vi "Configure Tare.vi"(8 "error in (no error)":errorcluster, 9 "Tare Value [g]":dbl, 10 "Set Value (F:Tare with current value)":bool, 11 "VISA resource name":refnum<visa-resource-name>) -> (0 "error out":errorcluster, 3 "VISA resource name out":refnum<visa-resource-name>)   [LabVIEW 2017, in "RadWag balances and scales.lvlib"]
doc: "Configures tare for the balance with current or given weight."
uses:
  <instrlib>/Radwag Balances and Scales/Public/RadWag balances and scales.lvlib
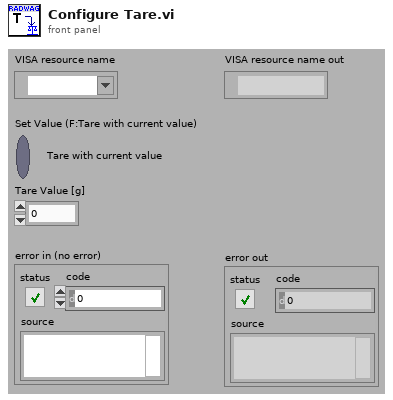
[diagram p1: front panel]
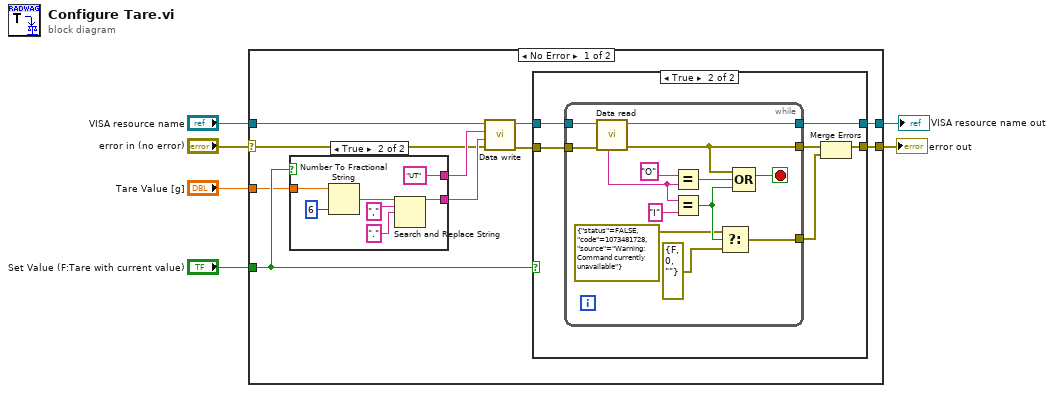
[diagram p0: block diagram]
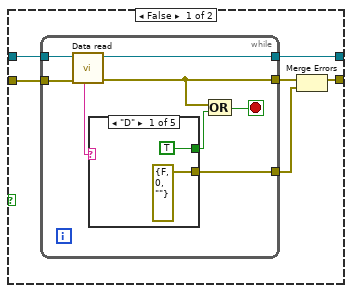
[diagram p2: hidden frame]
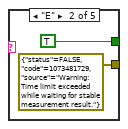
[diagram p3: hidden frame]
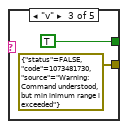
[diagram p4: hidden frame]
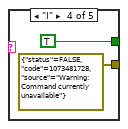
[diagram p5: hidden frame]
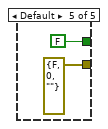
[diagram p6: hidden frame]
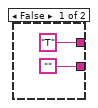
[diagram p7: hidden frame]
diagram:
  n1 = case shown="No Error" "error in (no error)" {
    selector: "error in (no error)" -> [w7 w69]
    tunnel: "VISA resource name" -> [w16 w70]
    tunnel: [w14 w70] -> w5
    tunnel: "Set Value (F:Tare with current value)" -> [w10 _]
    tunnel: [w9 w69] -> w3
    tunnel: "Tare Value [g]" -> [w8 _]
    frame No Error {
      n2 = case shown="True" w10 {
        tunnel: ["T" ("ID") "UT" ("ID")] -> w12
        tunnel: ["" w65] -> w11
        tunnel: w8 -> [_ w62]
        frame False {
        }
        frame True {
          n3 = Number To Fractional String(number=w62, precision (6)=i16 6) -> (F-format string=w66:string)  [unwired: 2 in]
          n4 = Search and Replace String(input string=w66, search string=",", replace string="." ("replace string (\"\")")) -> (result string=w65:string)  [unwired: 5 in, 3 out]
        }
      }
      n5 = call <instrlib>:"Data write.vi"("error in (no error)"=w7, "Parameter"=w11, "ID"=w12, "VISA resource name"=w16) -> ("error out"=w13:errorcluster, "VISA resource name out"=w15:refnum<visa-resource-name>)  [unwired: 6 in]
      n6 = case shown="True" w10 {
        tunnel: w15 -> [w22 w46]
        tunnel: [w20 w44] -> w14
        tunnel: w13 -> [w21 w45]
        tunnel: [w17 w42] -> w9
        frame False {
          n7 = while {
            tunnel: w22 -> [w30]
            tunnel: w21 -> [w29]
            tunnel: [w27] -> w20
            tunnel: [w26] -> w18
            tunnel: [w23] -> w19
            stop <- w28 stop-if-true
            n8 = call <instrlib>:"Data read.vi"("error in (no error)"=w29, "VISA resource name"=w30) -> ("error out"=w26:errorcluster, "VISA resource name out"=w27:refnum<visa-resource-name>, "Status"=w25:string)  [unwired: 3 in, 4 out]
            n9 = case shown="\"D\"" w25 {
              tunnel: [TRUE TRUE TRUE TRUE FALSE] -> w24
              tunnel: [errorcluster {"status"=FALSE, "code"=0, "source"=""} ("error constant") errorcluster {"status"=FALSE, "code"=1073481729, "source"="Warning: Time limit exceeded while waiting for stable measurement result."} ("t") errorcluster {"status"=FALSE, "code"=1073481730, "source"="Warning: Command understood, but min inimum range i exceeded"} ("t") errorcluster {"status"=FALSE, "code"=1073481728, "source"="Warning: Command currently unavailable"} ("t") errorcluster {"status"=FALSE, "code"=0, "source"=""} ("error constant")] -> w23
              frame "D" {
              }
              frame "E" {
              }
              frame "v" {
              }
              frame "I" {
              }
              frame Default {
              }
            }
            n10 = Compound Arithmetic op=OR(w26, w24) -> (w28:bool)
          }
          n11 = Merge Errors(w18, w19) -> (w17:errorcluster)
        }
        frame True {
          n12 = while {
            tunnel: w46 -> [w59]
            tunnel: [w54] -> w44
            tunnel: w45 -> [w55]
            tunnel: [w53] -> w43
            tunnel: [w48] -> w41
            stop <- w56 stop-if-true
            n13 = call <instrlib>:"Data read.vi"("error in (no error)"=w55, "VISA resource name"=w59) -> ("error out"=w53:errorcluster, "VISA resource name out"=w54:refnum<visa-resource-name>, "Status"=w57:string)  [unwired: 3 in, 4 out]
            n14 = Equal?(x="O", y=w57) -> (x = y?=w52:bool)
            n15 = Equal?(x=w57, y="I") -> (x = y?=w50:bool)
            n16 = Select(t=errorcluster {"status"=FALSE, "code"=1073481728, "source"="Warning: Command currently unavailable"}, s=w50, f=errorcluster {"status"=FALSE, "code"=0, "source"=""} ("error constant")) -> (s? t:f=w48:errorcluster)
            n17 = Compound Arithmetic op=OR(w53, w52, w50) -> (w56:bool)
          }
          n18 = Merge Errors(w43, w41) -> (w42:errorcluster)
        }
      }
    }
    frame Error {
    }
  }
  "VISA resource name out" <- w5
  "error out" <- w3
